vi "DataLogging_v2_TEST.vi"   [LabVIEW 2017]
uses:
  5409d957-8133-4fe8-ac06-cafa88ae112a.vi
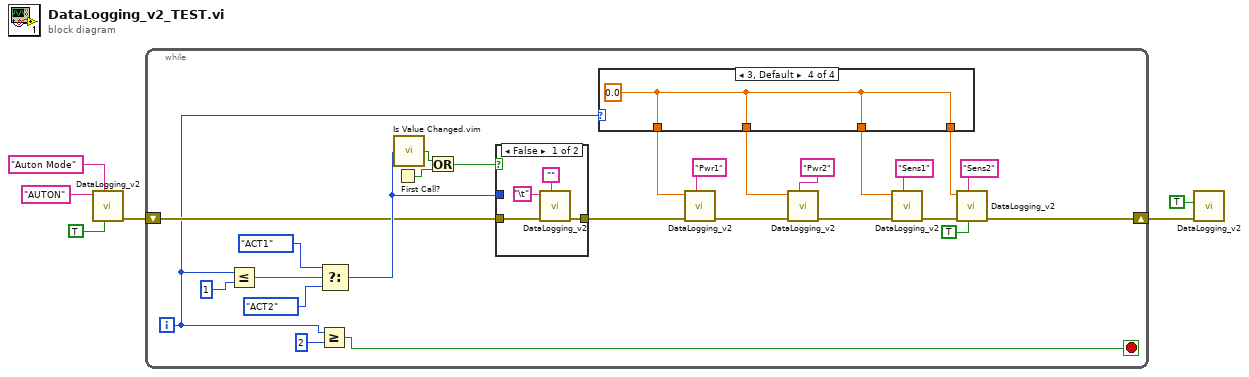
[diagram p0: block diagram]
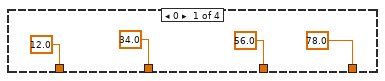
[diagram p2: hidden frame]
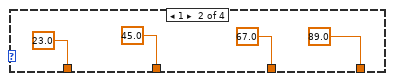
[diagram p3: hidden frame]
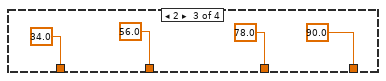
[diagram p4: hidden frame]
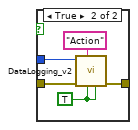
[diagram p5: hidden frame]
diagram:
  n1 = call "DataLogging_v2.vi"("New Line?"=TRUE, "Name"="Auton Mode", "Variant In"="AUTON" ("Name")) -> ("error out"=w4:errorcluster)  [unwired: 7 in, 1 out]
  n2 = while {
    shift-right: [w13] -> w3
    shift-left: w4 -> [w18]
    i -> [w12]
    stop <- w20 stop-if-true
    n3 = Less Or Equal?(x=w12, y=1 ("x")) -> (x <= y?=w25:bool)
    n4 = Greater Or Equal?(x=w12, y=2) -> (x >= y?=w20:bool)
    n5 = Select(t=enum16{"ACT1", "ACT2"}."ACT1", s=w25, f=enum16{"ACT1", "ACT2"}."ACT2") -> (s? t:f=w19:enum16{"ACT1", "ACT2"})
    n6 = First Call?() -> (First Call?: T/F=w28:bool)
    n7 = call "Is Value Changed.vim"("value"=w19) -> ("changed or first call?"=w27:bool)
    n8 = Or(x=w27, y=w28) -> (x .or. y?=w26:bool)
    n9 = case shown="False" w26 {
      tunnel: w19 -> [_ w53]
      tunnel: [w48 w52] -> w17
      tunnel: w18 -> [w47 w50]
      frame False {
        n10 = call "DataLogging_v2.vi"("Name"="", "error in (no error)"=w47, "Variant In"="\t") -> ("error out"=w48:errorcluster)  [unwired: 7 in, 1 out]
      }
      frame True {
        w51 = TRUE ("New Line?")
        n11 = call "DataLogging_v2.vi"("Tab?"=w51, "New Line?"=w51, "Name"="Action", "error in (no error)"=w50, "Variant In"=w53) -> ("error out"=w52:errorcluster)  [unwired: 5 in, 1 out]
      }
    }
    n12 = case shown="3, Default" w12 {
      tunnel: [12.0 23.0 34.0 w45] -> w11
      tunnel: [34.0 45.0 56.0 w45] -> w10
      tunnel: [56.0 67.0 78.0 w45] -> w9
      tunnel: [78.0 89.0 90.0 w45] -> w8
      frame 0 {
      }
      frame 1 {
      }
      frame 2 {
      }
      frame 3, Default {
        w45 = 0.0
      }
    }
    n13 = call "DataLogging_v2.vi"("Name"="Pwr1", "error in (no error)"=w17, "Variant In"=w11) -> ("error out"=w16:errorcluster)  [unwired: 7 in, 1 out]
    n14 = call "DataLogging_v2.vi"("Name"="Pwr2", "error in (no error)"=w16, "Variant In"=w10) -> ("error out"=w15:errorcluster)  [unwired: 7 in, 1 out]
    n15 = call "DataLogging_v2.vi"("Name"="Sens1", "error in (no error)"=w15, "Variant In"=w9) -> ("error out"=w14:errorcluster)  [unwired: 7 in, 1 out]
    n16 = call "DataLogging_v2.vi"("New Line?"=TRUE, "Name"="Sens2", "error in (no error)"=w14, "Variant In"=w8) -> ("error out"=w13:errorcluster)  [unwired: 6 in, 1 out]
  }
  n17 = call "DataLogging_v2.vi"("error in (no error)"=w3, "WriteToFile?"=TRUE) -> ()  [unwired: 8 in, 2 out]
